vi "Generate Unique Header.vi"(8 "error in":errorcluster, 11 "PAS Cell Data in":refnum<class "PAS Cell Data.lvclass">) -> (0 "error out":errorcluster, 2 "Header":string[](array[string]), 3 "PAS Cell Data out":refnum<class "PAS Cell Data.lvclass">)   [LabVIEW 2016, in "PAS Library.lvlib" / "PAS Cell Data.lvclass"]
uses:
  PAS Cell Data.lvclass
  C:/Program Files (x86)/National Instruments/LabVIEW 2016/vi.lib/MSR Consulting, LLC/General Reuse/Data/Data.lvclass
  Data/Data.lvclass/Data.ctl
  Data/Read Data ID.vi
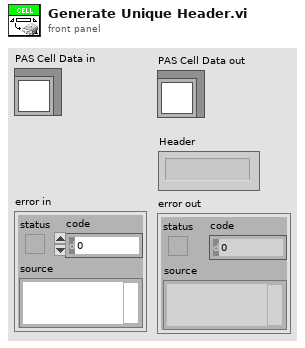
[diagram p1: front panel]
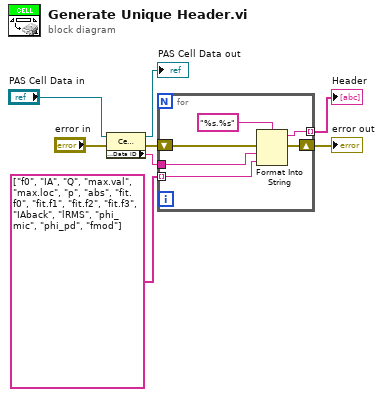
[diagram p0: block diagram]
diagram:
  n1 = property class="Cell Data"(reference="PAS Cell Data in", error in="error in") -> (reference out=→"PAS Cell Data out":refnum<class "PAS Cell Data.lvclass">, error out=w2:errorcluster, "Accessors:Data ID"=w4:string)
  n2 = for {
    tunnel: string[] ["f0", "IA", "Q", "max.val", "max.loc", "p", "abs", "fit.f0", "fit.f1", "fit.f2", "fit.f3", "IAback", "lRMS", "phi_mic", "phi_pd", "fmod"] -> [w14] mode=indexing
    tunnel: [w12] -> w7 mode=indexing
    tunnel: w4 -> [w11]
    shift-right: [w9] -> w1
    shift-left: w2 -> [w10]
    n3 = Format Into String(format string="%s.%s", error in=w10, w11, w14) -> (resulting string=w12:string, error out=w9:errorcluster)  [unwired: 1 in]
  }
  "error out" <- w1
  "Header" <- w7
